vi "base64decode.vi"(4 "Error In":errorcluster, 7 "string in (base64-encoded)":string) -> (0 "Error Out":errorcluster, 3 "string out (decoded)":string)   [LabVIEW 2015, in "Data Manipulation.lvlib"]
uses:
  Data Manipulation.lvlib
  <vilib>/Utility/error.llb/Error Cluster From Error Code.vi
  <vilib>/ErrorRing/Error Ring.xnode
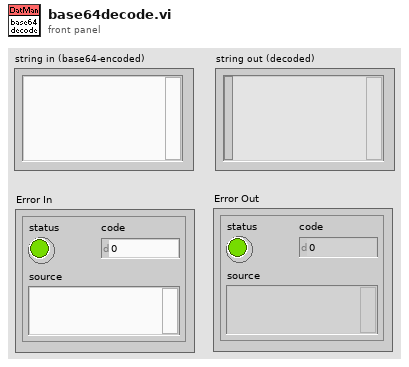
[diagram p1: front panel]
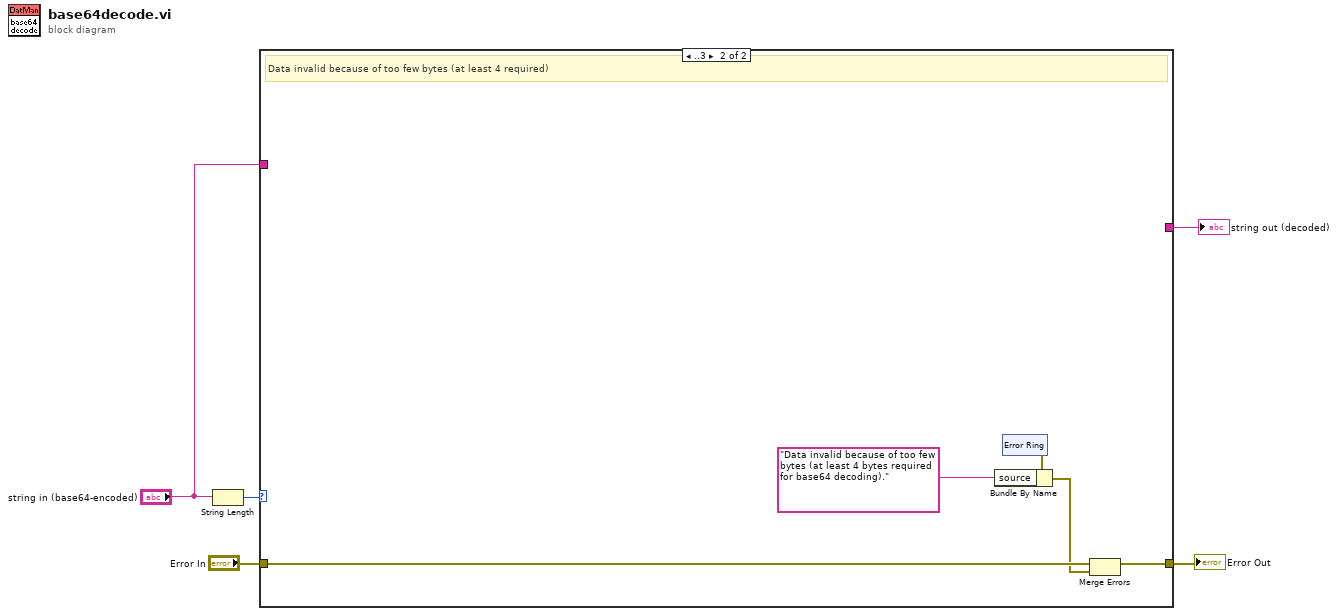
[diagram p0: block diagram]
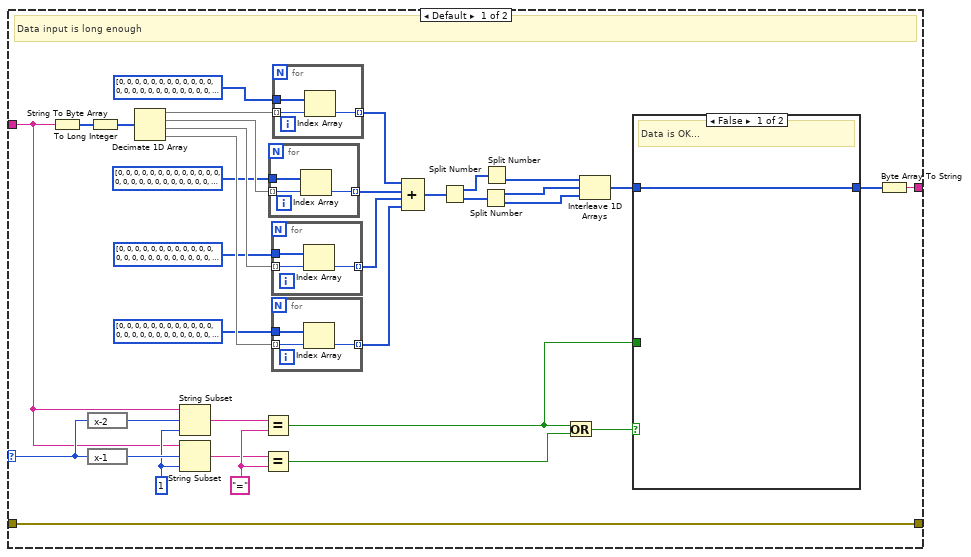
[diagram p2: hidden frame]
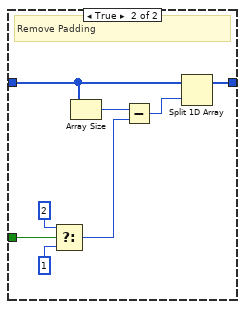
[diagram p3: hidden frame]
diagram:
  n1 = String Length(string="string in (base64-encoded)") -> (length=w2:i32)
  n2 = case shown="..3" w2 {
    selector: w2 -> [w9 _]
    tunnel: [w40 ""] -> w3
    tunnel: [w19 w66] -> w4
    tunnel: "Error In" -> [w19 w65]
    tunnel: "string in (base64-encoded)" -> [w8 _]
    frame Default {
      w15 = "="
      w11 = 1 ("length (rest)")
      # "Data input is long enough"
      n3 = String To Byte Array(string=w8) -> (unsigned byte array=w18:u8[])
      n4 = expression code="x-2"(w9) -> (w10:i32)
      n5 = expression code="x-1"(w9) -> (w12:i32)
      n6 = To Long Integer(number=w18) -> (32bit integer=w17:i32[])
      n7 = Decimate 1D Array(w17) -> (w29:i32[], w39:i32[], w30:i32[], w28:i32[])
      n8 = String Subset(string=w8, offset (0)=w10, length (rest)=w11) -> (substring=w13:string)
      n9 = String Subset(string=w8, offset (0)=w12, length (rest)=w11) -> (substring=w14:string)
      n10 = Equal?(x=w13, y=w15) -> (x = y?=w6:bool)
      n11 = Equal?(x=w14, y=w15) -> (x = y?=w16:bool)
      n12 = for {
        tunnel: w39 -> [w57] mode=indexing
        tunnel: u32[] [0, 0, 0, 0, 0, 0, 0, 0, 0, 0, 0, 0, 0, 0, 0, 0, 0, 0, 0, 0, 0, 0, 0, 0, 0, 0, 0, 0, 0, 0, 0, 0, 0, 0, 0, 0, 0, 0, 0, 0, 0, 0, 0, 253952, 0, 0, 0, 258048, 212992, 217088, 221184, 225280, 229376, 233472, 237568, 241664, 245760, 249856, 0, 0, 0, 0, 0, 0, 0, 0, 4096, 8192, 12288, 16384, 20480, 24576, 28672, 32768, 36864, 40960, 45056, 49152, 53248, 57344, 61440, 65536, 69632, 73728, 77824, 81920, 86016, 90112, 94208, 98304, 102400, 0, 0, 0, 0, 0, 0, 106496, 110592, 114688, 118784, 122880, 126976, 131072, 135168, 139264, 143360, 147456, 151552, 155648, 159744, 163840, 167936, 172032, 176128, 180224, 184320, 188416, 192512, 196608, 200704, 204800, 208896, 0, 0, 0, 0, 0, 0, 0, 0, 0, 0, 0, 0, 0, 0, 0, 0, 0, 0, 0, 0, 0, 0, 0, 0, 0, 0, 0, 0, 0, 0, 0, 0, 0, 0, 0, 0, 0, 0, 0, 0, 0, 0, 0, 0, 0, 0, 0, 0, 0, 0, 0, 0, 0, 0, 0, 0, 0, 0, 0, 0, 0, 0, 0, 0, 0, 0, 0, 0, 0, 0, 0, 0, 0, 0, 0, 0, 0, 0, 0, 0, 0, 0, 0, 0, 0, 0, 0, 0, 0, 0, 0, 0, 0, 0, 0, 0, 0, 0, 0, 0, 0, 0, 0, 0, 0, 0, 0, 0, 0, 0, 0, 0, 0, 0, 0, 0, 0, 0, 0, 0, 0, 0, 0, 0, 0, 0, 0, 0, 0, 0, 0, 0, 0] ("array 3") -> [w58]
        tunnel: [w56] -> w37 mode=indexing
        n13 = Index Array(array=w58, index=w57) -> (element=w56:u32)
      }
      n14 = for {
        tunnel: u32[] [0, 0, 0, 0, 0, 0, 0, 0, 0, 0, 0, 0, 0, 0, 0, 0, 0, 0, 0, 0, 0, 0, 0, 0, 0, 0, 0, 0, 0, 0, 0, 0, 0, 0, 0, 0, 0, 0, 0, 0, 0, 0, 0, 3968, 0, 0, 0, 4032, 3328, 3392, 3456, 3520, 3584, 3648, 3712, 3776, 3840, 3904, 0, 0, 0, 4278190080, 0, 0, 0, 0, 64, 128, 192, 256, 320, 384, 448, 512, 576, 640, 704, 768, 832, 896, 960, 1024, 1088, 1152, 1216, 1280, 1344, 1408, 1472, 1536, 1600, 0, 0, 0, 0, 0, 0, 1664, 1728, 1792, 1856, 1920, 1984, 2048, 2112, 2176, 2240, 2304, 2368, 2432, 2496, 2560, 2624, 2688, 2752, 2816, 2880, 2944, 3008, 3072, 3136, 3200, 3264, 0, 0, 0, 0, 0, 0, 0, 0, 0, 0, 0, 0, 0, 0, 0, 0, 0, 0, 0, 0, 0, 0, 0, 0, 0, 0, 0, 0, 0, 0, 0, 0, 0, 0, 0, 0, 0, 0, 0, 0, 0, 0, 0, 0, 0, 0, 0, 0, 0, 0, 0, 0, 0, 0, 0, 0, 0, 0, 0, 0, 0, 0, 0, 0, 0, 0, 0, 0, 0, 0, 0, 0, 0, 0, 0, 0, 0, 0, 0, 0, 0, 0, 0, 0, 0, 0, 0, 0, 0, 0, 0, 0, 0, 0, 0, 0, 0, 0, 0, 0, 0, 0, 0, 0, 0, 0, 0, 0, 0, 0, 0, 0, 0, 0, 0, 0, 0, 0, 0, 0, 0, 0, 0, 0, 0, 0, 0, 0, 0, 0, 0, 0, 0] ("array 2") -> [w55]
        tunnel: [w54] -> w23 mode=indexing
        tunnel: w30 -> [w53] mode=indexing
        n15 = Index Array(array=w55, index=w53) -> (element=w54:u32)
      }
      n16 = for {
        tunnel: u32[] [0, 0, 0, 0, 0, 0, 0, 0, 0, 0, 0, 0, 0, 0, 0, 0, 0, 0, 0, 0, 0, 0, 0, 0, 0, 0, 0, 0, 0, 0, 0, 0, 0, 0, 0, 0, 0, 0, 0, 0, 0, 0, 0, 62, 0, 0, 0, 63, 52, 53, 54, 55, 56, 57, 58, 59, 60, 61, 0, 0, 0, 4278190080, 0, 0, 0, 0, 1, 2, 3, 4, 5, 6, 7, 8, 9, 10, 11, 12, 13, 14, 15, 16, 17, 18, 19, 20, 21, 22, 23, 24, 25, 0, 0, 0, 0, 0, 0, 26, 27, 28, 29, 30, 31, 32, 33, 34, 35, 36, 37, 38, 39, 40, 41, 42, 43, 44, 45, 46, 47, 48, 49, 50, 51, 0, 0, 0, 0, 0, 0, 0, 0, 0, 0, 0, 0, 0, 0, 0, 0, 0, 0, 0, 0, 0, 0, 0, 0, 0, 0, 0, 0, 0, 0, 0, 0, 0, 0, 0, 0, 0, 0, 0, 0, 0, 0, 0, 0, 0, 0, 0, 0, 0, 0, 0, 0, 0, 0, 0, 0, 0, 0, 0, 0, 0, 0, 0, 0, 0, 0, 0, 0, 0, 0, 0, 0, 0, 0, 0, 0, 0, 0, 0, 0, 0, 0, 0, 0, 0, 0, 0, 0, 0, 0, 0, 0, 0, 0, 0, 0, 0, 0, 0, 0, 0, 0, 0, 0, 0, 0, 0, 0, 0, 0, 0, 0, 0, 0, 0, 0, 0, 0, 0, 0, 0, 0, 0, 0, 0, 0, 0, 0, 0, 0, 0, 0, 0] ("Array") -> [w52]
        tunnel: [w51] -> w22 mode=indexing
        tunnel: w28 -> [w50] mode=indexing
        n17 = Index Array(array=w52, index=w50) -> (element=w51:u32)
      }
      n18 = for {
        tunnel: w29 -> [w60] mode=indexing
        tunnel: u32[] [0, 0, 0, 0, 0, 0, 0, 0, 0, 0, 0, 0, 0, 0, 0, 0, 0, 0, 0, 0, 0, 0, 0, 0, 0, 0, 0, 0, 0, 0, 0, 0, 0, 0, 0, 0, 0, 0, 0, 0, 0, 0, 0, 16252928, 0, 0, 0, 16515072, 13631488, 13893632, 14155776, 14417920, 14680064, 14942208, 15204352, 15466496, 15728640, 15990784, 0, 0, 0, 0, 0, 0, 0, 0, 262144, 524288, 786432, 1048576, 1310720, 1572864, 1835008, 2097152, 2359296, 2621440, 2883584, 3145728, 3407872, 3670016, 3932160, 4194304, 4456448, 4718592, 4980736, 5242880, 5505024, 5767168, 6029312, 6291456, 6553600, 0, 0, 0, 0, 0, 0, 6815744, 7077888, 7340032, 7602176, 7864320, 8126464, 8388608, 8650752, 8912896, 9175040, 9437184, 9699328, 9961472, 10223616, 10485760, 10747904, 11010048, 11272192, 11534336, 11796480, 12058624, 12320768, 12582912, 12845056, 13107200, 13369344, 0, 0, 0, 0, 0, 0, 0, 0, 0, 0, 0, 0, 0, 0, 0, 0, 0, 0, 0, 0, 0, 0, 0, 0, 0, 0, 0, 0, 0, 0, 0, 0, 0, 0, 0, 0, 0, 0, 0, 0, 0, 0, 0, 0, 0, 0, 0, 0, 0, 0, 0, 0, 0, 0, 0, 0, 0, 0, 0, 0, 0, 0, 0, 0, 0, 0, 0, 0, 0, 0, 0, 0, 0, 0, 0, 0, 0, 0, 0, 0, 0, 0, 0, 0, 0, 0, 0, 0, 0, 0, 0, 0, 0, 0, 0, 0, 0, 0, 0, 0, 0, 0, 0, 0, 0, 0, 0, 0, 0, 0, 0, 0, 0, 0, 0, 0, 0, 0, 0, 0, 0, 0, 0, 0, 0, 0, 0, 0, 0, 0, 0, 0, 0] ("array 4") -> [w61]
        tunnel: [w59] -> w38 mode=indexing
        n19 = Index Array(array=w61, index=w60) -> (element=w59:u32)
      }
      n20 = Compound Arithmetic op=ADD(w38, w37, w23, w22) -> (w35:u32[])
      n21 = Split Number(x=w35) -> (hi(x)=w36:u16[], lo(x)=w34:u16[])
      n22 = Split Number(x=w34) -> (hi(x)=w32:u8[], lo(x)=w33:u8[])
      n23 = Split Number(x=w36) -> (lo(x)=w31:u8[])  [unwired: 1 out]
      n24 = Or(x=w6, y=w16) -> (x .or. y?=w7:bool)
      n25 = Interleave 1D Arrays(w31, w32, w33) -> (w21:u8[])
      n26 = case shown="False" w7 {
        tunnel: w21 -> [w41 w46]
        tunnel: [w41 w48] -> w20
        tunnel: w6 -> [_ w43]
        frame False {
          # "Data is OK..."
        }
        frame True {
          # "Remove Padding"
          n27 = Select(t=2, s=w43, f=1) -> (s? t:f=w42:i32)
          n28 = Array Size(array=w46) -> (size(s)=w47:i32)
          n29 = Subtract(x=w47, y=w42) -> (x-y=w49:i32)
          n30 = Split 1D Array(array=w46, index=w49) -> (first subarray=w48:u8[])  [unwired: 1 out]
        }
      }
      n31 = Byte Array To String(unsigned byte array=w20) -> (string=w40:string)
    }
    frame ..3 {
      # "Data invalid because of too few bytes (at least 4 required)"
      n32 = xnode "Error Ring"() -> ("error out"=w64:errorcluster)
      n33 = Bundle By Name(cluster=w64, "source"="Data invalid because of too few bytes (at least 4 bytes required for base64 decoding).") -> (w63:errorcluster)
      n34 = Merge Errors(w65, w63) -> (w66:errorcluster)
    }
  }
  "Error Out" <- w4
  "string out (decoded)" <- w3
